vi "Configure.vi"(8 "error in (no error)":errorcluster, 11 "ServiceManager in":refnum<class "ServiceManager.lvclass">) -> (0 "error out":errorcluster, 2 "cancelled?":bool, 3 "ServiceManager out":refnum<class "ServiceManager.lvclass">)   [LabVIEW 2012, in "ServiceManager.lvclass"]
uses:
  ServiceManager.lvclass
  settings_enum.ctl
  <vilib>/Utility/miscctls.llb/LVPointTypeDef.ctl
  ServiceManager.lvclass/ServiceManager.ctl
  Murmex/LabVIEW/Murmex/Murmex/Murmex.lvclass
panel:
  in  "button:delete_setting":bool
  in  "button:add_setting":bool
  in  "setting":T1
  in  "button:add path manually":bool
  in  "button:edit path":bool
  in  "button:delete path":bool
  in  "button:add path":bool
  in  "search paths":i32(listbox)
  in  "button:edit":bool
  in  "button:delete":bool
  in  "button:parent":bool
  in  "button:cancel":bool
  in  "button:ok":bool
  in  "button:add":bool
  in  "components":i32(listbox)
  # "Configure ServiceManager"
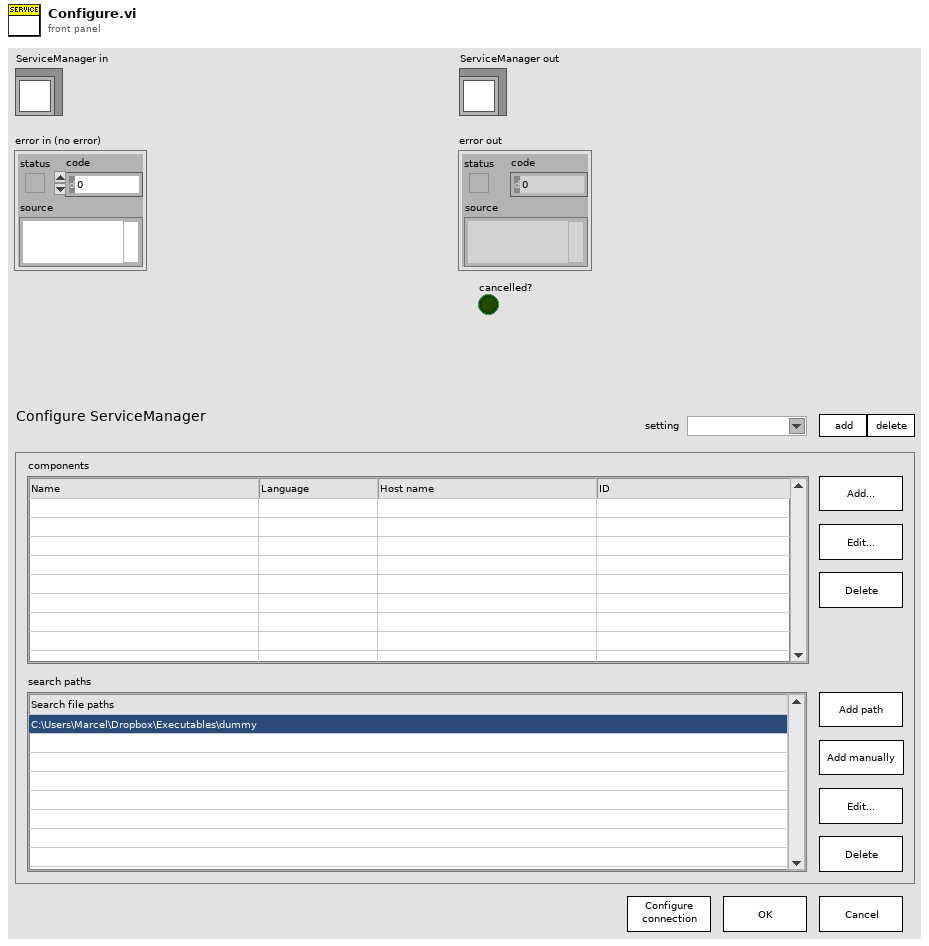
[diagram p1: front panel]
types:
  T1 = typedef "ServiceManager.lvclass/settings_enum.ctl" = string
  T2 = typedef "LVPointTypeDef.ctl" = cluster{"Horizontal":i16, "Vertical":i16}
  T3 = typedef "ServiceManager.lvclass/configuration_enum.ctl" = string
  T4 = typedef "Murmex.lvlib/Murmex.lvclass/component_specification_cluster.ctl" = cluster{"name":string, "language":string, "host name":string, "id":string}
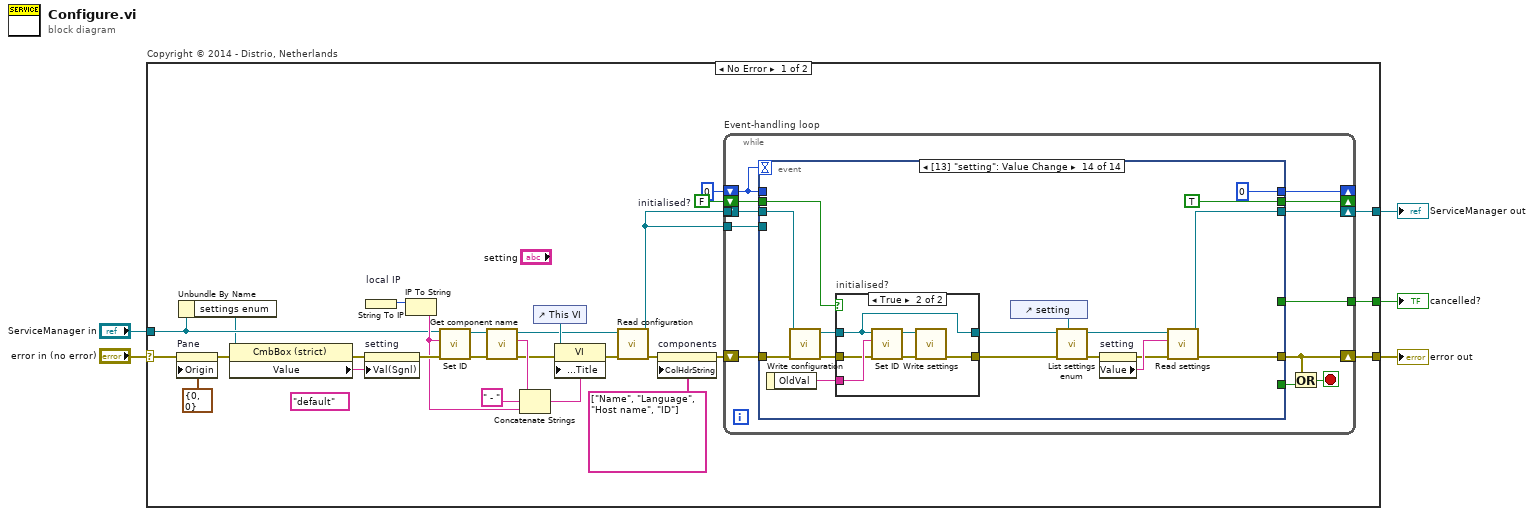
[diagram p0: block diagram]
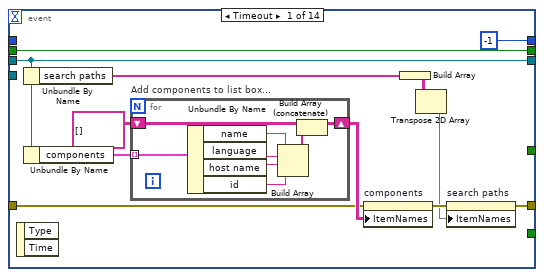
[diagram p2: hidden frame]
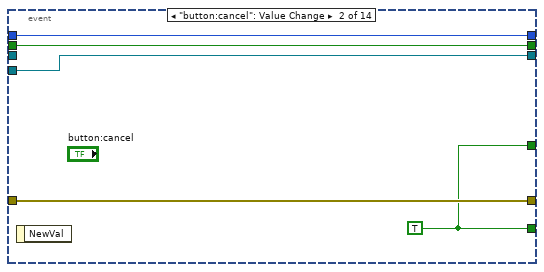
[diagram p3: hidden frame]
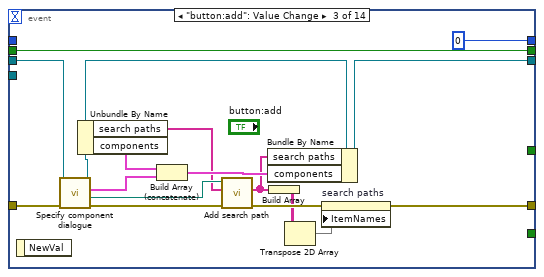
[diagram p4: hidden frame]
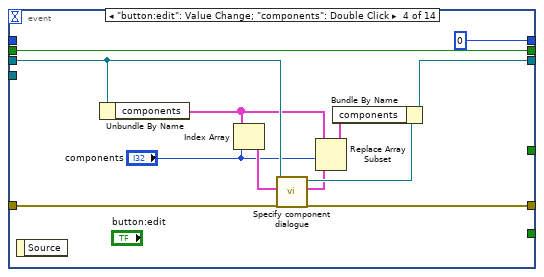
[diagram p5: hidden frame]
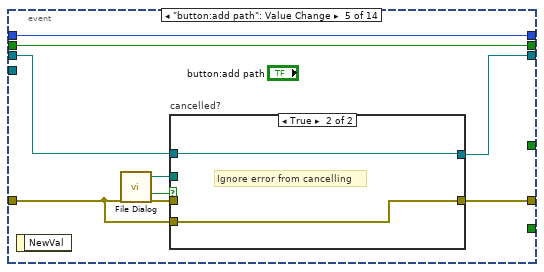
[diagram p6: hidden frame]
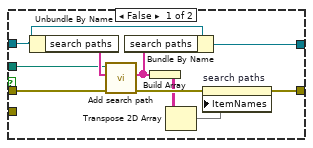
[diagram p7: hidden frame]
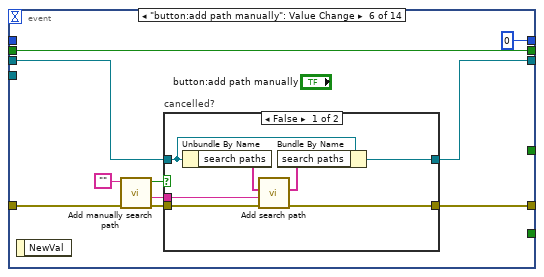
[diagram p8: hidden frame]
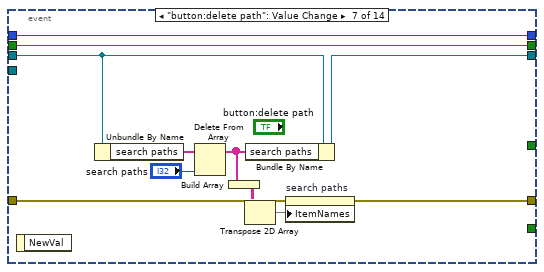
[diagram p10: hidden frame]
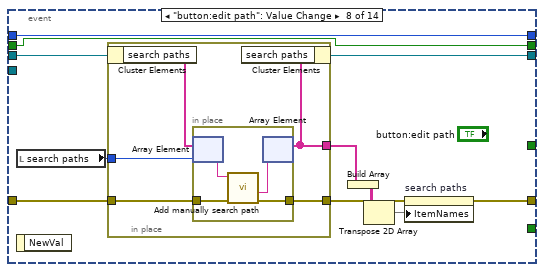
[diagram p11: hidden frame]
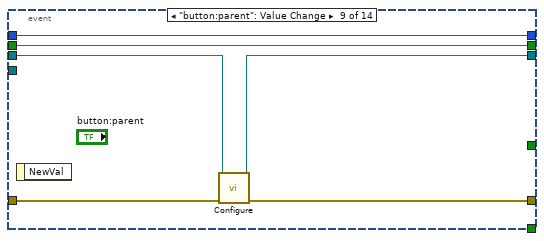
[diagram p12: hidden frame]
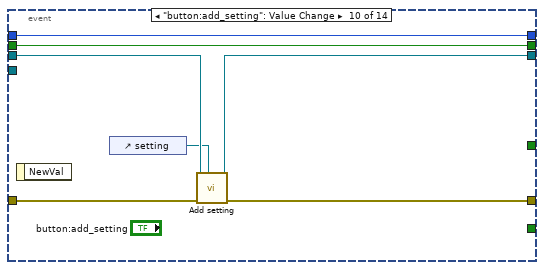
[diagram p13: hidden frame]
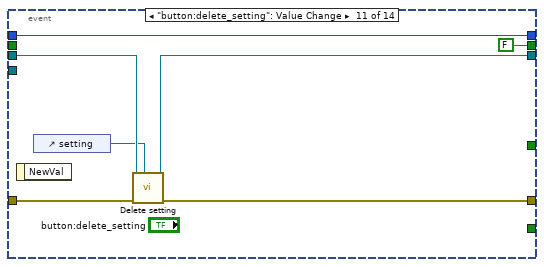
[diagram p14: hidden frame]
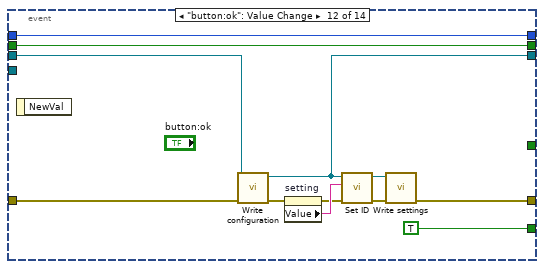
[diagram p15: hidden frame]
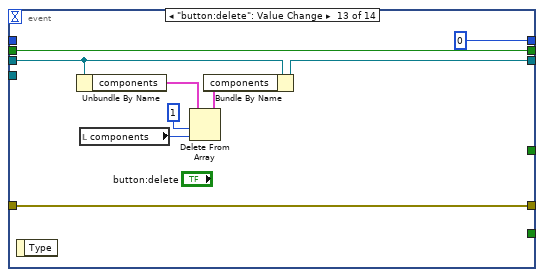
[diagram p16: hidden frame]
diagram:
  n1 = case "Copyright © 2014 - Distrio, Netherlands" shown="No Error" "error in (no error)" {
    selector: "error in (no error)" -> [w23 w238]
    tunnel: "ServiceManager in" -> [w10 w239]
    tunnel: [w32 w239] -> w4
    tunnel: [w31 w238] -> w3
    tunnel: [w21 _] -> w1
    frame No Error {
      (unwired) "default"
      w20 = FALSE  # initialised?
      n2 = property on="Pane" class="Pane"(error in=w23, "Origin"=T2 {"Horizontal"=0, "Vertical"=0}) -> (error out=w7:errorcluster)  [unwired: 1 in, 1 out]
      n3 = Unbundle By Name(w10) -> ("settings enum"=w9:refnum<vi>)
      n4 = property class="CmbBox (strict)"(reference=w9, error in=w7) -> (error out=w6:errorcluster, "Value"=w8:T3)  [unwired: 1 out]
      n5 = property on="setting" class="CmbBox (strict)"(error in=w6, "Val(Sgnl)"=w8) -> (error out=w22:errorcluster)  [unwired: 1 in, 1 out]
      n6 = String To IP "local IP"() -> (0:w30:u32)  [unwired: 1 in]
      n7 = IP To String(2:w30) -> (0:w14:string)  [unwired: 1 in]
      n8 = call "Set ID.vi"("error in (no error)"=w22, "id"=w14, "Murmex in"=w10) -> ("error out"=w17:errorcluster, "Murmex out"=w28:refnum<class "ServiceManager.lvclass">)  [unwired: 7 in]
      n9 = call "Get component name.vi"("error in (no error)"=w17, "Murmex in"=w28) -> ("error out"=w12:errorcluster, "component name"=w16:string, "Murmex out"=w18:refnum<class "ServiceManager.lvclass">)  [unwired: 7 in]
      n10 = Concatenate Strings(w16, " - " ("string"), w14) -> (w13:string)
      n11 = control-ref of="This VI"() -> (w19:refnum<vi>)
      n12 = property class="VI"(reference=w19, error in=w12, "Front Panel.Title"=w13) -> (error out=w11:errorcluster)  [unwired: 1 out]
      n13 = call "Read configuration.vi"("error in (no error)"=w11, "Murmex in"=w18) -> ("error out"=w26:errorcluster, "Murmex out"=w29:refnum<class "ServiceManager.lvclass">)  [unwired: 7 in, 1 out]
      n14 = property on="components" class="MCListbox (strict)"(error in=w26, "ColHdrString"=string[] ["Name", "Language", "Host name", "ID"] ("Column Header Strings[]")) -> (error out=w25:errorcluster)  [unwired: 1 in, 1 out]
      n15 = while "Event-handling loop" {
        shift-right: [w45] -> w31
        shift-left: w25 -> [w46]
        shift-right: [w39] -> w32
        shift-left: w29 -> [w42]
        shift-right: [w40] -> _
        shift-left: 0 -> [w41]
        tunnel: w29 -> [w38]
        tunnel: w29 -> [w37]
        tunnel: [w36] -> w21
        shift-right: [w34] -> _
        shift-left: w20 -> [w35]
        stop <- w43 stop-if-true
        n16 = event shown="[13] \"setting\": Value Change" {
          selector: _ -> [_ _ _ _ _ _ _ _ _ _ _ _ _ _]
          dyn-events: _ -> [_ _ _ _ _ _ _ _ _ _ _ _ _ _]
          timeout: w41 -> [_ _ _ _ _ _ _ _ _ _ _ _ _ _]
          tunnel: w46 -> [w53 w71 w84 w100 w101 w128 w149 w154 w176 w183 w189 w201 w212 w223]
          tunnel: [w51 w71 w80 w99 w108 w131 w148 w157 w175 w182 w188 w193 w212 w217] -> w45
          tunnel: [_ w68 _ _ _ _ _ _ _ _ _ TRUE _ _] -> w44
          tunnel: w42 -> [w54 _ w83 w96 w103 w130 w145 w156 w174 w181 w190 w192 w211 w226]
          tunnel: [-1 w70 0 0 w109 0 w151 w162 w177 w184 w191 w202 0 0] -> w40
          tunnel: w41 -> [_ w70 _ _ w109 _ w151 w162 w177 w184 w191 w202 _ _]
          tunnel: [w54 w69 w85 w97 w107 w129 w144 w155 w173 w180 w187 w195 w210 w213] -> w39
          tunnel: w38 -> [_ _ _ _ _ _ _ _ _ _ _ _ _ _]
          tunnel: w37 -> [_ w69 _ _ _ _ _ _ _ _ _ _ _ _]
          tunnel: [_ w68 _ _ _ _ _ _ _ _ _ _ _ _] -> w36
          tunnel: w35 -> [w47 w67 w72 w90 w106 w123 w141 w152 w172 w179 _ w199 w205 w219]
          tunnel: [w47 w67 w72 w90 w106 w123 w141 w152 w172 w179 FALSE ("initialised?") w199 w205 TRUE ("initialised?")] -> w34
          event Timeout {
            n17 = event-data() -> ()  [unwired: 1 in, 2 out]
            n18 = Unbundle By Name(w54) -> ("search paths"=w50:string[])
            n19 = Unbundle By Name(w54) -> ("components"=w58:T4[])
            n20 = for "Add components to list box..." {
              tunnel: w58 -> [w66] mode=indexing
              shift-right: [w59] -> w55
              shift-left: string[][] [] -> [w60]
              n21 = Unbundle By Name(w66) -> ("name"=w65:string, "language"=w62:string, "host name"=w63:string, "id"=w64:string)
              n22 = Build Array(w65, w62, w63, w64) -> (w61:string[])
              n23 = Build Array (concatenate)(w60, w61) -> (w59:string[][])
            }
            n24 = property on="components" class="MCListbox (strict)"(error in=w53, "ItemNames"=w55) -> (error out=w52:errorcluster)  [unwired: 1 in, 1 out]
            n25 = Build Array(w50) -> (w49:string[][])
            n26 = Transpose 2D Array(2D array=w49) -> (transposed array=w48:string[][])
            n27 = property on="search paths" class="MCListbox (strict)"(error in=w52, "ItemNames"=w48) -> (error out=w51:errorcluster)  [unwired: 1 in, 1 out]
          }
          event "button:cancel": Value Change {
            w68 = TRUE
            n28 = event-data() -> ()  [unwired: 1 in, 1 out]
          }
          event "button:add": Value Change {
            n29 = event-data() -> ()  [unwired: 1 in, 1 out]
            n30 = call "Specify component dialogue.vi"("error in (no error)"=w84, "ServiceManager in"=w83) -> ("error out"=w77:errorcluster, "path out"=w78:path, "component specification out"=w81:T4, "ServiceManager out"=w82:refnum<class "ServiceManager.lvclass">)  [unwired: 6 in]
            n31 = Unbundle By Name(w82) -> ("search paths"=w74:string[], "components"=w87:T4[])
            n32 = Build Array (concatenate)(w87, w81) -> (w86:T4[])
            n33 = call "Add search path.vi"("error in (no error)"=w77, "array in"=w74, "path in"=w78) -> ("error out"=w76:errorcluster, "array out"=w73:string[])  [unwired: 7 in]
            n34 = Bundle By Name(cluster=w82, "search paths"=w73, "components"=w86) -> (w85:refnum<class "ServiceManager.lvclass">)
            n35 = Build Array(w73) -> (w75:string[][])
            n36 = Transpose 2D Array(2D array=w75) -> (transposed array=w79:string[][])
            n37 = property on="search paths" class="MCListbox (strict)"(error in=w76, "ItemNames"=w79) -> (error out=w80:errorcluster)  [unwired: 1 in, 1 out]
          }
          event "button:edit": Value Change; "components": Double Click {
            n38 = event-data() -> ()  [unwired: 1 in, 1 out]
            n39 = Unbundle By Name(w96) -> ("components"=w93:T4[])
            n40 = Index Array(array=w93, index="components") -> (element=w91:T4)
            n41 = call "Specify component dialogue.vi"("error in (no error)"=w100, "component specification in"=w91, "ServiceManager in"=w96) -> ("error out"=w99:errorcluster, "component specification out"=w94:T4, "ServiceManager out"=w95:refnum<class "ServiceManager.lvclass">)  [unwired: 5 in, 1 out]
            n42 = Replace Array Subset(array=w93, new element=w94, index="components") -> (w92:T4[])
            n43 = Bundle By Name(cluster=w95, "components"=w92) -> (w97:refnum<class "ServiceManager.lvclass">)
          }
          event "button:add path": Value Change {
            n44 = event-data() -> ()  [unwired: 1 in, 1 out]
            n45 = call "File Dialog"("error in"=w101) -> ("selected path"=w105:path, "cancelled"=w102:bool, "error out"=w104:errorcluster)  [unwired: 11 in, 1 out]
            n46 = case "cancelled?" shown="True" w102 {
              tunnel: [w116 w120] -> w108
              tunnel: w103 -> [w113 w121]
              tunnel: [w112 w121] -> w107
              tunnel: w105 -> [w111 _]
              tunnel: w104 -> [w110 _]
              tunnel: w101 -> [_ w120]
              frame False {
                n47 = Unbundle By Name(w113) -> ("search paths"=w115:string[])
                n48 = call "Add search path.vi"("error in (no error)"=w110, "array in"=w115, "path in"=w111) -> ("error out"=w118:errorcluster, "array out"=w114:string[])  [unwired: 7 in]
                n49 = Bundle By Name(cluster=w113, "search paths"=w114) -> (w112:refnum<class "ServiceManager.lvclass">)
                n50 = Build Array(w114) -> (w117:string[][])
                n51 = Transpose 2D Array(2D array=w117) -> (transposed array=w119:string[][])
                n52 = property on="search paths" class="MCListbox (strict)"(error in=w118, "ItemNames"=w119) -> (error out=w116:errorcluster)  [unwired: 1 in, 1 out]
              }
              frame True {
                # "Ignore error from cancelling"
              }
            }
          }
          event "button:add path manually": Value Change {
            n53 = event-data() -> ()  [unwired: 1 in, 1 out]
            n54 = call "Add manually search path.vi"("error in (no error)"=w128, "string in"="") -> ("error out"=w127:errorcluster, "manual path out"=w126:string, "cancelled?"=w125:bool)  [unwired: 7 in]
            n55 = case "cancelled?" shown="False" w125 {
              tunnel: [w132 w139] -> w131
              tunnel: w130 -> [w136 w140]
              tunnel: [w135 w140] -> w129
              tunnel: w127 -> [w134 w139]
              tunnel: w126 -> [w133 _]
              frame False {
                n56 = Unbundle By Name(w136) -> ("search paths"=w138:string[])
                n57 = call "Add search path.vi"("error in (no error)"=w134, "path in"=w133, "array in"=w138) -> ("error out"=w132:errorcluster, "array out"=w137:string[])  [unwired: 7 in]
                n58 = Bundle By Name(cluster=w136, "search paths"=w137) -> (w135:refnum<class "ServiceManager.lvclass">)
              }
              frame True {
              }
            }
          }
          event "button:delete path": Value Change {
            n59 = event-data() -> ()  [unwired: 1 in, 1 out]
            n60 = Unbundle By Name(w145) -> ("search paths"=w143:string[])
            n61 = Delete From Array(array=w143, index="search paths") -> (array with subset deleted=w142:string[])  [unwired: 1 in, 1 out]
            n62 = Build Array(w142) -> (w147:string[][])
            n63 = Transpose 2D Array(2D array=w147) -> (transposed array=w146:string[][])
            n64 = Bundle By Name(cluster=w145, "search paths"=w142) -> (w144:refnum<class "ServiceManager.lvclass">)
            n65 = property on="search paths" class="MCListbox (strict)"(error in=w149, "ItemNames"=w146) -> (error out=w148:errorcluster)  [unwired: 1 in, 1 out]
          }
          event "button:edit path": Value Change {
            n66 = local read "search paths"() -> (w161:i32)
            n67 = event-data() -> ()  [unwired: 1 in, 1 out]
            n68 = in-place {
              in-place-border: w161 -> [w167]
              in-place-border: [w165] -> w158
              in-place-border: w154 -> [w164]
              in-place-border: [w163] -> w153
              n69 = in-place-cluster #1(w156) -> ("search paths"=w166:string[])
              n70 = in-place {
                in-place-border: w164 -> [w169]
                in-place-border: [w168] -> w163
                n71 = in-place-array #2(w166, w167) -> (w171:string)
                n72 = call "Add manually search path.vi"("error in (no error)"=w169, "string in"=w171) -> ("error out"=w168:errorcluster, "manual path out"=w170:string)  [unwired: 7 in, 1 out]
                n73 = in-place-array #2(w170) -> (w165:string[])  [unwired: 1 out]
              }
              n74 = in-place-cluster #1("search paths"=w165) -> (w155:refnum<class "ServiceManager.lvclass">)
            }
            n75 = Build Array(w158) -> (w160:string[][])
            n76 = Transpose 2D Array(2D array=w160) -> (transposed array=w159:string[][])
            n77 = property on="search paths" class="MCListbox (strict)"(error in=w153, "ItemNames"=w159) -> (error out=w157:errorcluster)  [unwired: 1 in, 1 out]
          }
          event "button:parent": Value Change {
            n78 = event-data() -> ()  [unwired: 1 in, 1 out]
            n79 = call-parent "Configure.vi"("error in (no error)"=w176, "Murmex in"=w174) -> ("error out"=w175:errorcluster, "Murmex out"=w173:refnum<class "ServiceManager.lvclass">)  [unwired: 7 in, 1 out]
          }
          event "button:add_setting": Value Change {
            n80 = event-data() -> ()  [unwired: 1 in, 1 out]
            n81 = control-ref of="setting"() -> (w178:refnum<vi>)
            n82 = call-dynamic "Add setting.vi"("setting reference"=w178, "error in (no error)"=w183, "ServiceManager in"=w181) -> ("error out"=w182:errorcluster, "ServiceManager out"=w180:refnum<class "ServiceManager.lvclass">)  [unwired: 7 in]
          }
          event "button:delete_setting": Value Change {
            n83 = event-data() -> ()  [unwired: 1 in, 1 out]
            n84 = control-ref of="setting"() -> (w185:refnum<vi>)
            n85 = call-dynamic "Delete setting.vi"("setting reference"=w185, "error in (no error)"=w189, "ServiceManager in"=w190) -> ("error out"=w188:errorcluster, "ServiceManager out"=w187:refnum<class "ServiceManager.lvclass">)  [unwired: 7 in]
          }
          event "button:ok": Value Change {
            n86 = event-data() -> ()  [unwired: 1 in, 1 out]
            n87 = call "Write configuration.vi"("error in (no error)"=w201, "Murmex in"=w192) -> ("error out"=w200:errorcluster, "Murmex out"=w195:refnum<class "ServiceManager.lvclass">)  [unwired: 8 in]
            n88 = property on="setting" class="CmbBox (strict)"(error in=w200) -> (error out=w194:errorcluster, "Value"=w196:T1)  [unwired: 1 in, 1 out]
            n89 = call "Set ID.vi"("error in (no error)"=w194, "id"=w196, "Murmex in"=w195) -> ("error out"=w197:errorcluster, "Murmex out"=w198:refnum<class "ServiceManager.lvclass">)  [unwired: 7 in]
            n90 = call-dynamic "Write settings.vi"("error in (no error)"=w197, "Murmex in"=w198) -> ("error out"=w193:errorcluster)  [unwired: 7 in, 2 out]
          }
          event "button:delete": Value Change {
            n91 = event-data() -> ()  [unwired: 1 in, 1 out]
            n92 = Unbundle By Name(w211) -> ("components"=w209:T4[])
            n93 = local read "components"() -> (w204:i32)
            n94 = Delete From Array(array=w209, length=1, index=w204) -> (array with subset deleted=w208:T4[])  [unwired: 1 out]
            n95 = Bundle By Name(cluster=w211, "components"=w208) -> (w210:refnum<class "ServiceManager.lvclass">)
          }
          event Value Change {
            n96 = event-data() -> ("OldVal"=w221:T1)  [unwired: 1 in]
            n97 = call "Write configuration.vi"("error in (no error)"=w223, "Murmex in"=w226) -> ("error out"=w224:errorcluster, "Murmex out"=w227:refnum<class "ServiceManager.lvclass">)  [unwired: 8 in]
            n98 = case "initialised?" shown="True" w219 {
              tunnel: w227 -> [w231 w232]
              tunnel: [w231 w232] -> w225
              tunnel: w224 -> [w230 w236]
              tunnel: [w230 w233] -> w222
              tunnel: w221 -> [_ w237]
              frame False {
              }
              frame True {
                n99 = call "Set ID.vi"("error in (no error)"=w236, "id"=w237, "Murmex in"=w232) -> ("error out"=w234:errorcluster, "Murmex out"=w235:refnum<class "ServiceManager.lvclass">)  [unwired: 7 in]
                n100 = call-dynamic "Write settings.vi"("error in (no error)"=w234, "Murmex in"=w235) -> ("error out"=w233:errorcluster)  [unwired: 7 in, 2 out]
              }
            }
            n101 = control-ref of="setting"() -> (w218:refnum<vi>)
            n102 = call-dynamic "List settings enum.vi"("setting enum reference"=w218, "error in (no error)"=w222, "ServiceManager in"=w225) -> ("error out"=w229:errorcluster, "ServiceManager out"=w214:refnum<class "ServiceManager.lvclass">)  [unwired: 7 in]
            n103 = property on="setting" class="CmbBox (strict)"(error in=w229) -> (error out=w215:errorcluster, "Value"=w216:T1)  [unwired: 1 in, 1 out]
            n104 = call-dynamic "Read settings.vi"("error in (no error)"=w215, "settings name"=w216, "Murmex in"=w214) -> ("error out"=w217:errorcluster, "Murmex out"=w213:refnum<class "ServiceManager.lvclass">)  [unwired: 5 in, 2 out]
          }
        }
        n105 = Or(x=w45, y=w44) -> (x .or. y?=w43:bool)
      }
    }
    frame Error {
    }
  }
  "error out" <- w3
  "ServiceManager out" <- w4
  "cancelled?" <- w1
